vi "TT_CODE.vi"(8 "errin":errorcluster, 11 "pathin":path) -> (0 "error out":errorcluster, 3 "Delay calculé":string)   [LabVIEW 2020]
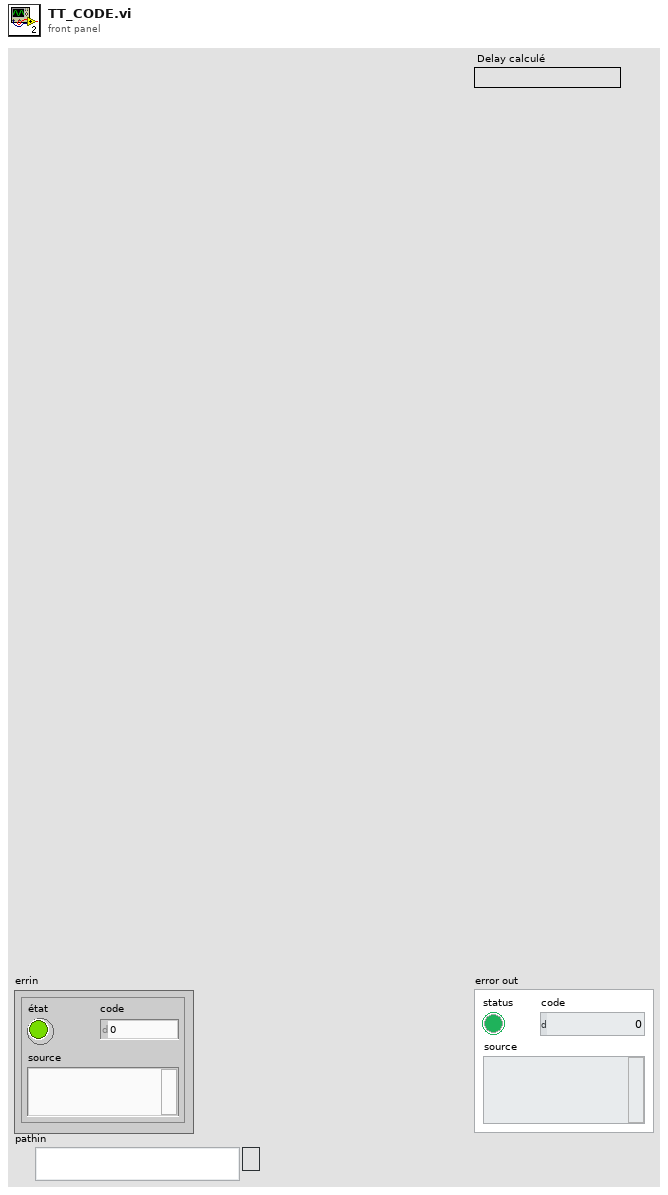
[diagram p1: front panel]
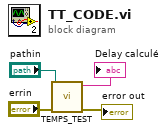
[diagram p0: block diagram]
diagram:
  n1 = call <userlib>:"TEMPS_TEST.vi"("errin"="errin", "pathin"="pathin") -> ("error out"=→"error out":errorcluster, "Delay calculé"=→"Delay calculé":string)  [unwired: 8 in]
